vi "MoveAbs.vi"(8 "error in":errorcluster, 9 "Axis":i32, 10 "Position":dbl, 11 "VISA resource":refnum<visa-resource-name>) -> (0 "error out":errorcluster)   [LabVIEW 2014, in "GRBLMotionCore.lvlib"]
uses:
  <instrlib>/GRBL/GrblMotionCore.lvlib
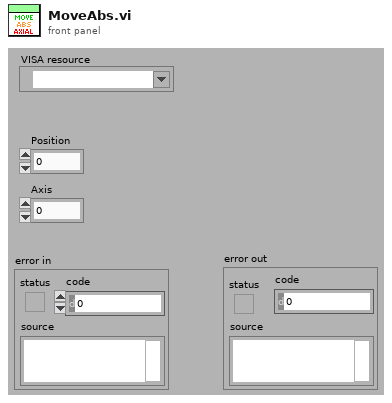
[diagram p1: front panel]
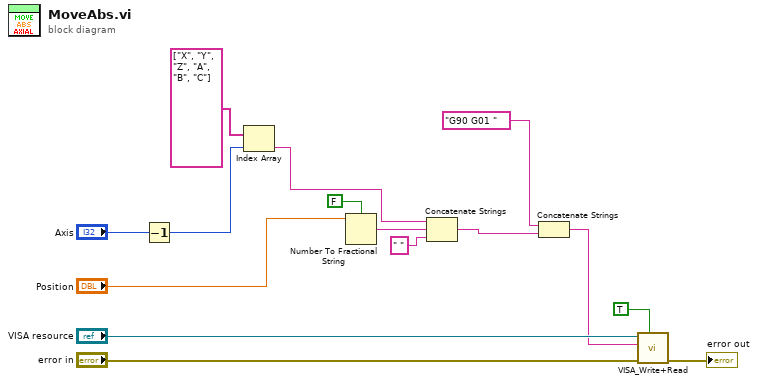
[diagram p0: block diagram]
diagram:
  n1 = Decrement(x="Axis") -> (x-1=w7:i32)
  n2 = Index Array(array=string[] ["X", "Y", "Z", "A", "B", "C"], index=w7) -> (element=w5:string)
  n3 = Number To Fractional String(use system decimal point (T)=FALSE, number="Position") -> (F-format string=w3:string)  [unwired: 2 in]
  n4 = Concatenate Strings(w5, w3, " " ("string")) -> (w10:string)
  n5 = Concatenate Strings("G90 G01 ", w10) -> (w11:string)
  n6 = call <instrlib>:"VISA_Write+Read.vi"("Read?"=TRUE, "error in (no error)"="error in", "Write Buffer"=w11, "VISA resource name"="VISA resource") -> ("error out"=→"error out":errorcluster)  [unwired: 5 in, 2 out]
